vi "Set 2D Array Double Complex.vi"(5 "use temporary file? (F)":bool, 8 "error in":errorcluster, 9 "value":cdb[][](array[numeric]), 10 "variable name":string, 11 "GOLPI ref. in":T1={"pipe handle"={"lv_proc.dll file path"=path "", "process instance handle"=[], "debug mode"=FALSE, "debug data"=[]}, "fast read timeout [ms]"=500, "fast read settle time [ms]"=10, "fast read to multiple [ms]"=1, "max elements per input line"=100, "slow read timeout [ms]"=5000, "stdin double format specifier"="%_16e", "max elements per stdout output column"=100, "console mode bitstream"=FALSE, "bitstream first read timeout [ms]"=1000, "bitstream read timeout [ms]"=50, "struct transfer possible"=FALSE, "matlab mode"=FALSE}) -> (0 "error out":errorcluster, 3 "GOLPI ref. out":T1={"pipe handle"={"lv_proc.dll file path"=path "", "process instance handle"=[], "debug mode"=FALSE, "debug data"=[]}, "fast read timeout [ms]"=500, "fast read settle time [ms]"=10, "fast read to multiple [ms]"=1, "max elements per input line"=100, "slow read timeout [ms]"=5000, "stdin double format specifier"="%_16e", "max elements per stdout output column"=100, "console mode bitstream"=FALSE, "bitstream first read timeout [ms]"=1000, "bitstream read timeout [ms]"=50, "struct transfer possible"=FALSE, "matlab mode"=FALSE})   [LabVIEW 2020, in "GOLPI library.lvlib"]
doc: "Part of polymorph Set Variable.vi"
uses:
  GOLPI library.lvlib
  GOLPI reference Type Def.ctl
  Pipe Handle.ctl
  LV Process library.lvlib
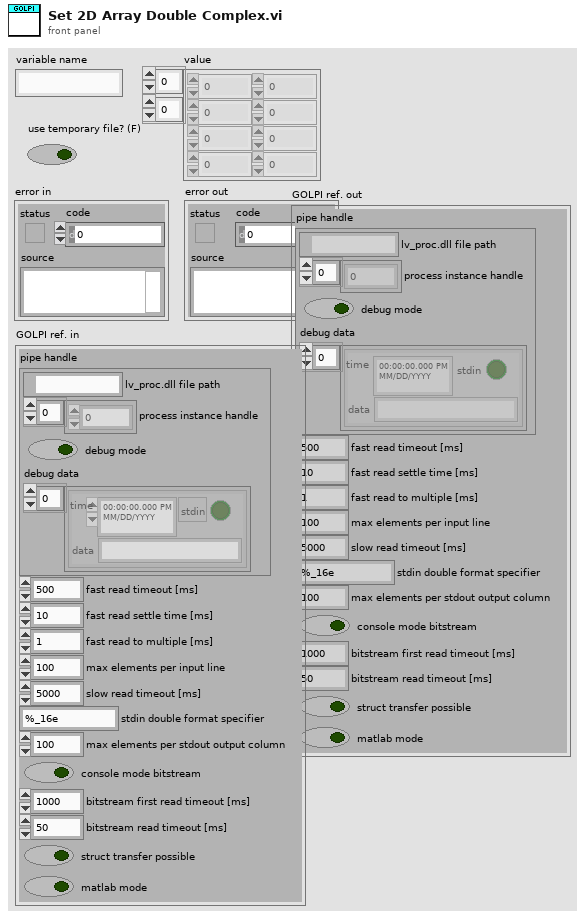
[diagram p1: front panel]
types:
  T1 = typedef "GOLPI library.lvlib/GOLPI reference Type Def.ctl" = cluster{"pipe handle":T2, "fast read timeout [ms]":u32, "fast read settle time [ms]":u32, "fast read to multiple [ms]":u32, "max elements per input line":u32, "slow read timeout [ms]":u32, "stdin double format specifier":string, "max elements per stdout output column":u32, "console mode bitstream":bool, "bitstream first read timeout [ms]":u32, "bitstream read timeout [ms]":u32, "struct transfer possible":bool, "matlab mode":bool}
  T2 = typedef "LV Process library.lvlib/Pipe Handle.ctl" = cluster{"lv_proc.dll file path":path, "process instance handle":u32[], "debug mode":bool, "debug data":cluster{"time":timestamp, "stdin":bool, "data":string}[]}
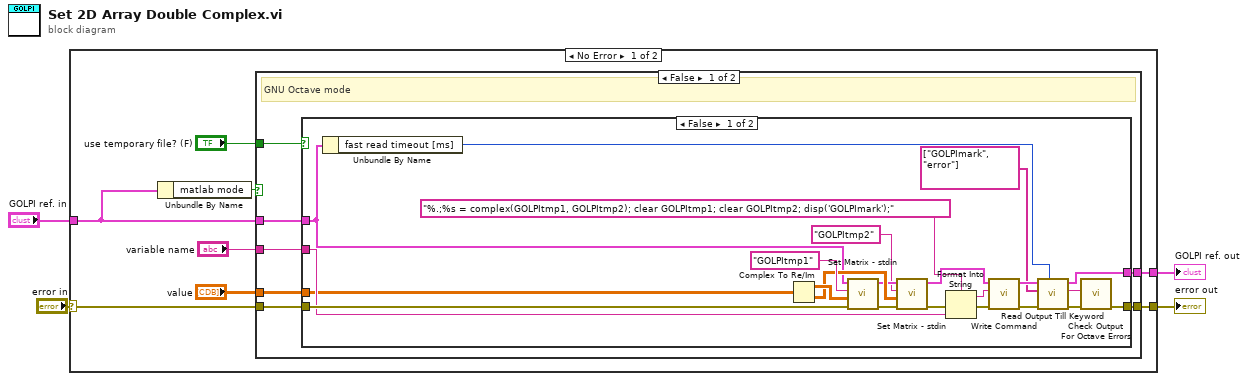
[diagram p0: block diagram]
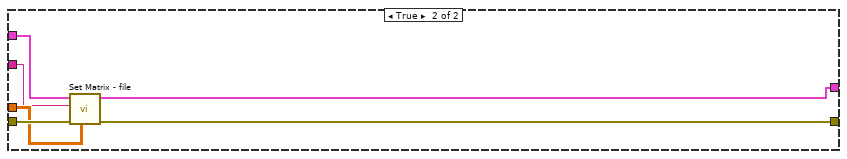
[diagram p2: hidden frame]
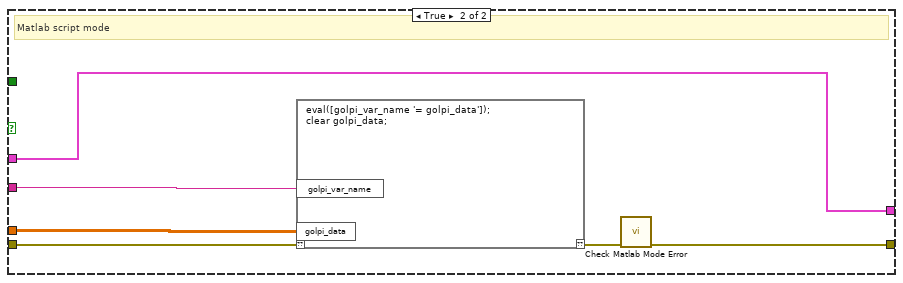
[diagram p3: hidden frame]
diagram:
  n1 = case shown="No Error" "error in" {
    selector: "error in" -> [w12 w56]
    tunnel: [w10 w56] -> w4
    tunnel: "GOLPI ref. in" -> [w6 w55]
    tunnel: [w11 w55] -> w1
    frame No Error {
      n2 = Unbundle By Name(w6) -> ("matlab mode"=w5:bool)
      n3 = case shown="False" w5 {
        tunnel: w12 -> [w19 w54]
        tunnel: [w18 w51] -> w11
        tunnel: [w17 w49] -> w10
        tunnel: "variable name" -> [w16 w52]
        tunnel: w6 -> [w15 w51]
        tunnel: "use temporary file? (F)" -> [w14 _]
        tunnel: "value" -> [w13 w53]
        frame False {
          # "GNU Octave mode"
          n4 = case shown="False" w14 {
            tunnel: w19 -> [w42 w48]
            tunnel: [w32 w46] -> w18
            tunnel: [w29 w47] -> w17
            tunnel: w16 -> [w27 w43]
            tunnel: w15 -> [w22 w45]
            tunnel: w13 -> [w20 w44]
            frame False {
              n5 = Unbundle By Name(w22) -> ("fast read timeout [ms]"=w21:u32)
              n6 = Complex To Re/Im(x + iy=w20) -> (x=w41:dbl[][], y=w39:dbl[][])
              n7 = call "Set Matrix - stdin.vi"("error in"=w42, "value"=w41, "variable name"="GOLPItmp1", "GOLPI ref. in"=w22) -> ("error out"=w37:errorcluster, "GOLPI ref. out"=w38:T1)  [unwired: 6 in]
              n8 = call "Set Matrix - stdin.vi"("error in"=w37, "value"=w39, "variable name"="GOLPItmp2", "GOLPI ref. in"=w38) -> ("error out"=w26:errorcluster, "GOLPI ref. out"=w35:T1)  [unwired: 6 in]
              n9 = Format Into String(format string="%.;%s = complex(GOLPItmp1, GOLPItmp2); clear GOLPItmp1; clear GOLPItmp2; disp('GOLPImark');" ("command"), error in=w26, w27) -> (resulting string=w23:string, error out=w25:errorcluster)  [unwired: 1 in]
              n10 = call "Write Command.vi"("error in"=w25, "command"=w23, "GOLPI ref. in"=w35) -> ("error out"=w24:errorcluster, "GOLPI ref. out"=w34:T1)  [unwired: 7 in]
              n11 = call "Read Output Till Keyword.vi"("timeout [ms]"=w21, "error in"=w24, "keywords"=string[] ["GOLPImark", "error"], "GOLPI ref. in"=w34) -> ("error out"=w30:errorcluster, "read buffer"=w31:string, "GOLPI ref. out"=w32:T1)  [unwired: 4 in, 1 out]
              n12 = call "Check Output For Octave Errors.vi"("error in"=w30, "read buffer"=w31) -> ("error out"=w29:errorcluster)  [unwired: 9 in]
            }
            frame True {
              n13 = call "Set Matrix - file.vi"("cmplx double array"=w44, "error in (no error)"=w48, "variable name"=w43, "GOLPI ref. in"=w45) -> ("error out"=w47:errorcluster, "GOLPI ref. out"=w46:T1)  [unwired: 6 in]
            }
          }
        }
        frame True {
          # "Matlab script mode"
          n14 = script code="eval([golpi_var_name '= golpi_data']);\nclear golpi_data;"("??"=w54, "golpi_var_name"=w52, "golpi_data"=w53) -> ("??"=w50:errorcluster)
          n15 = call "Check Matlab Mode Error.vi"("error in"=w50) -> ("error out"=w49:errorcluster)  [unwired: 10 in]
        }
      }
    }
    frame Error {
    }
  }
  "error out" <- w4
  "GOLPI ref. out" <- w1
